vi "Constructor.vi"(8 "error in":errorcluster, 11 "Singleton Abstract":refnum<class "Singleton.lvclass">) -> (0 "error out":errorcluster, 3 "Singleton Abstract":refnum<class "Singleton.lvclass">)   [LabVIEW 2009, in "Singleton.lvclass"]
doc: "OVERRIDE VI\nPlaceholder for decendant sessions to initialize and set their default values"
uses:
  Singleton.lvclass
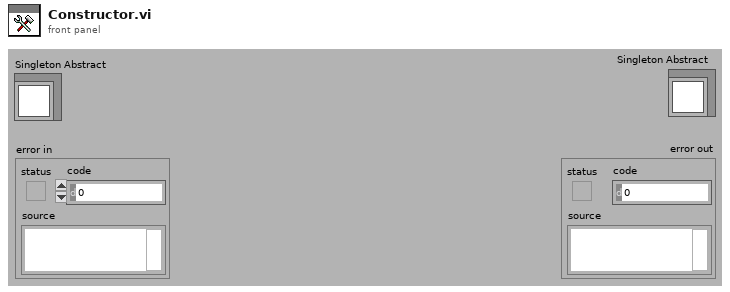
[diagram p1: front panel]
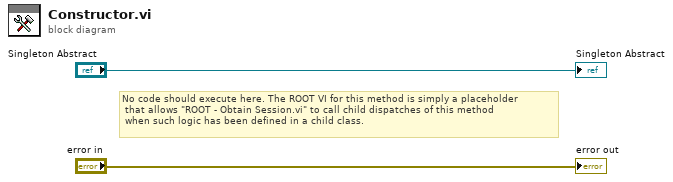
[diagram p0: block diagram]
diagram:
  # "No code should execute here. The ROOT VI for this method is simply a placeholder\n that allows \"ROOT - Obtain Session.vi\" to call child dispatches of this method\n when such logic has been defined in a child class."
  "error out" <- "error in"
  "Singleton Abstract" <- "Singleton Abstract"
